vi "Measurement Logic.vi"(8 "error in":errorcluster, 9 "measurement configuration":T2={"TDMS File Path"="", "TDMS Channels"=["", ""], "FGEN Resource Names"=["", ""], "TDMS Groups"=["", ""], "FGEN Waveform Names"=["", ""], "Export Marker0 From File?"=TRUE, "Waveform Sequence"=["", ""], "Loops Sequence"=[]}, 10 "measure call context in":refnum<class "Measure Call Context.lvclass">) -> (0 "error out":errorcluster, 1 "measurement results":T1, 2 "measure call context out":refnum<class "Measure Call Context.lvclass">)   [LabVIEW 2025, in "FGEN Arb Sequence Mode.lvclass"]
doc: "Contains the core logic for executing the measurement."
uses:
  FGEN Arb Sequence Mode.lvclass
  <vilib>/Plug-In SDKs/Measurements/Measure Call Context/Measure Call Context.lvclass
  Measurement Configuration.ctl
  Measurement Results.ctl
  71329b31-811e-493e-9c7a-fa078d8b0f92.vi
  71329b31-811e-493e-9c7a-fa078d8b0f92.vi/9a3a9ab8-4bd1-41e7-91e7-3b9acfe124d7.vi
  <vilib>/Utility/error.llb/Error Cluster From Error Code.vi
  <extravilib>/ChannelInstances/Event Messenger-bool/Instantiate.vi
  FGEN Arb Sequence Mode.lvclass/FGEN Arb Sequence Mode.ctl
  <vilib>/Plug-In SDKs/Clients/Session Management V1/Session Reservation/Session Reservation.lvclass
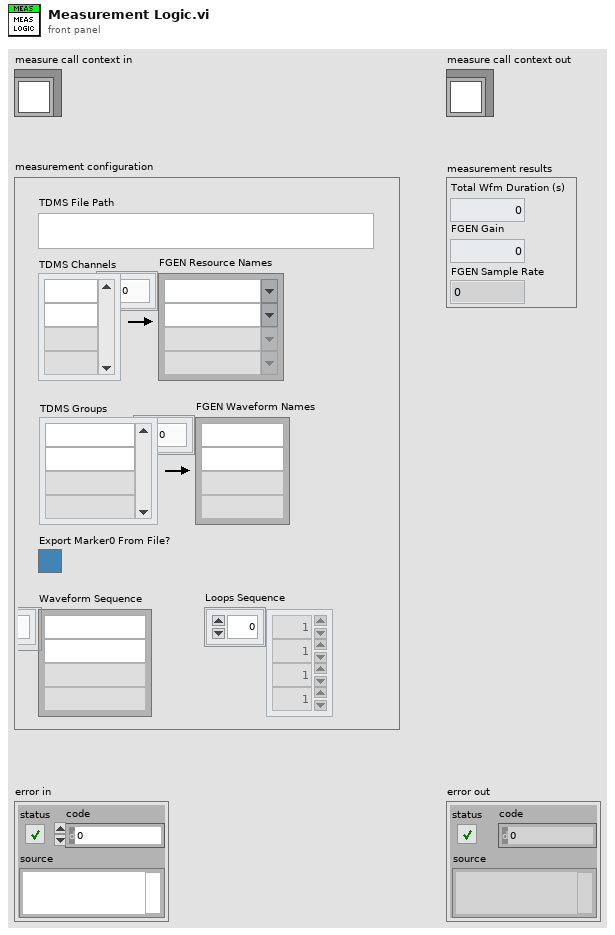
[diagram p1: front panel]
types:
  T1 = typedef "FGEN Arb Sequence Mode.lvclass/Measurement Results.ctl" = cluster{"Total Wfm Duration (s)":dbl, "FGEN Gain":dbl, "FGEN Sample Rate":dbl}
  T2 = typedef "FGEN Arb Sequence Mode.lvclass/Measurement Configuration.ctl" = cluster{"TDMS File Path":string, "TDMS Channels":string[], "FGEN Resource Names":string[], "TDMS Groups":string[], "FGEN Waveform Names":string[], "Export Marker0 From File?":bool, "Waveform Sequence":string[], "Loops Sequence":u32[]}
  T3 = cluster{"FGEN Channels":string[], "FGEN Gain":dbl, "FGEN Wfm Sequence":string[], "FGEN Loops Sequence":u32[], "FGEN Wfm Map":map{string, cluster{"Waveforms":waveform(dbl)[], "Markers":dbl}}, "Sample Rate":dbl}
  T4 = cluster{"FGEN Channel Mapping":string[][], "FGEN Wfm List":string[][]}
  T5 = cluster{"FGEN Channels":string[], "FGEN Gain":dbl, "FGEN Sample Rate":dbl, "FGEN Wfm Map":map{string, cluster{"Waveforms":waveform(dbl)[], "Markers":dbl}}}
  T6 = map{string, cluster{"Waveforms":waveform(dbl)[], "Markers":dbl}}
  T7 = cluster{"session reservation out":refnum<class "Session Reservation.lvclass">, "session":refnum<k15>}
  T8 = typedef "Event Messenger-bool.lvlib/))Channel.ctl" = refnum<queue>
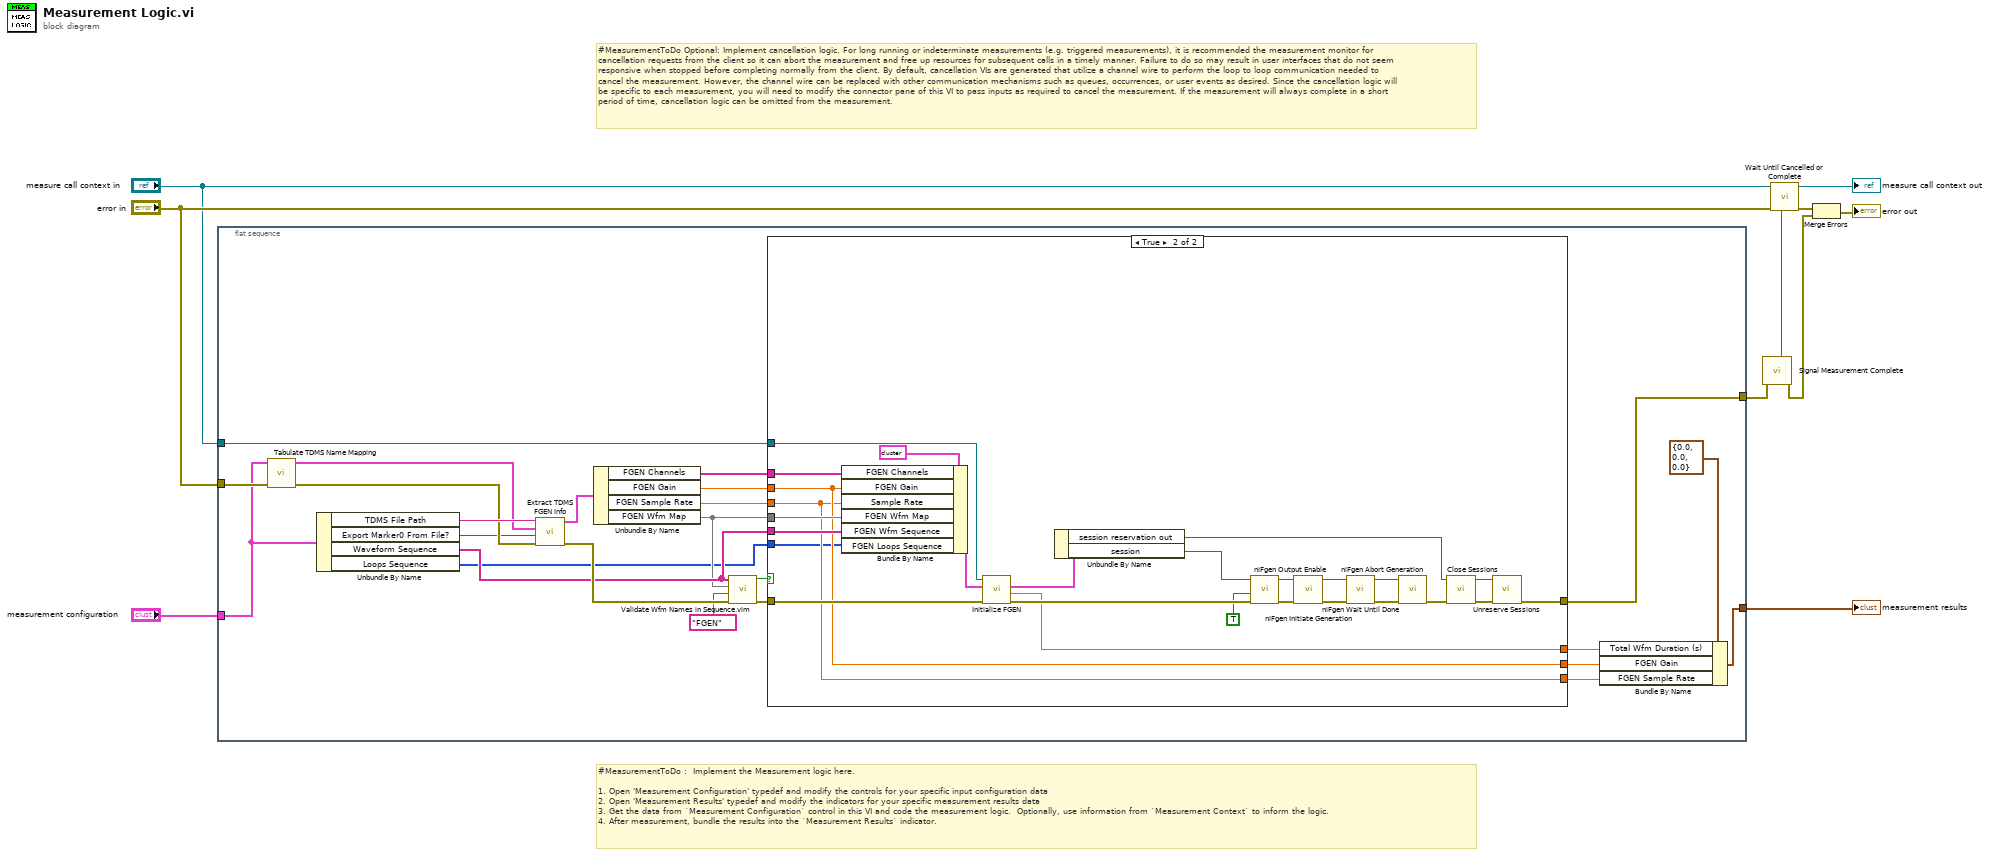
[diagram p0: block diagram]
diagram:
  # "#MeasurementToDo Optional: Implement cancellation logic. For long running or indeterminate measurements (e.g. triggered measurements), it is recommended the measurement monitor for cancellation requests from the client so it can abort the measurement and free up resources for subsequent calls in a timely manner. Failure to do so may result in user interfaces that do not seem responsive when stopped before completing normally from the client. By default, cancellation VIs are generated that utilize a channel wire to perform the loop to loop communication needed to cancel the measurement. However, the channel wire can be replaced with other communication mechanisms such as queues, occurrences, or user events as desired. Since the cancellation logic will be specific to each measurement, you will need to modify the connector pane of this VI to pass inputs as required to cancel the measurement. If the measurement will always complete in a short period of time, cancellation logic can be omitted from the measurement."
  # "#MeasurementToDo :  Implement the Measurement logic here.\n\n1. Open 'Measurement Configuration' typedef and modify the controls for your specific input configuration data\n2. Open 'Measurement Results' typedef and modify the indicators for your specific measurement results data\n3. Get the data from `Measurement Configuration` control in this VI and code the measurement logic.  Optionally, use information from `Measurement Context` to inform the logic.\n4. After measurement, bundle the results into the `Measurement Results` indicator."
  n1 = flat-sequence {
    tunnel: "measurement configuration" -> [w20]
    tunnel: [w33] -> w9
    tunnel: "error in" -> [w28]
    tunnel: [w15] -> w6
    tunnel: "measure call context in" -> [w23]
    frame #0 {
      n2 = call "Tabulate TDMS Name Mapping.vi"("error in"=w28, "measurement configuration"=w20) -> ("error out"=w30:errorcluster, "TDMS Name Mapping"=w31:T4)  [unwired: 8 in]
      n3 = Unbundle By Name(w20) -> ("TDMS File Path"=w32:string, "Export Marker0 From File?"=w27:bool, "Waveform Sequence"=w21:string[], "Loops Sequence"=w11:u32[])
      n4 = call "Extract TDMS FGEN Info.vi"("error in (no error)"=w30, "Export Marker0 From File?"=w27, "TDMS Name Mapping"=w31, "TDMS File Path"=w32) -> ("error out"=w29:errorcluster, "TDMS FGEN Info"=w25:T5)  [unwired: 6 in]
      n5 = Unbundle By Name(w25) -> ("FGEN Channels"=w22:string[], "FGEN Gain"=w17:dbl, "FGEN Sample Rate"=w16:dbl, "FGEN Wfm Map"=w19:T6)
      n6 = call "Validate Wfm Names in Sequence.vim"("error in"=w29, "Wfm Resource Type"="FGEN", "Wfm Map"=w19, "Wfm Sequence"=w21) -> ("error out"=w26:errorcluster, "All Waveform Name Valid?"=w14:bool)  [unwired: 6 in]
      n7 = case shown="True" w14 {
        tunnel: w26 -> [w35 w61]
        tunnel: w23 -> [_ w59]
        tunnel: w22 -> [_ w57]
        tunnel: w21 -> [_ w56]
        tunnel: w19 -> [_ w55]
        tunnel: [_ w53] -> w18
        tunnel: w17 -> [_ w40]
        tunnel: w16 -> [_ w39]
        tunnel: [w35 w46] -> w15
        tunnel: [_ w40] -> w13
        tunnel: [_ w39] -> w12
        tunnel: w11 -> [_ w36]
        frame False {
        }
        frame True {
          n8 = Bundle By Name(cluster=T3 {"FGEN Channels"=[], "FGEN Gain"=0.0, "FGEN Wfm Sequence"=[], "FGEN Loops Sequence"=[], "FGEN Wfm Map"={}, "Sample Rate"=0.0} ("FGEN Settings"), "FGEN Channels"=w57, "FGEN Gain"=w40, "Sample Rate"=w39, "FGEN Wfm Map"=w55, "FGEN Wfm Sequence"=w56, "FGEN Loops Sequence"=w36) -> (w58:T3)
          n9 = call "Initialize FGEN.vi"("error in (no error)"=w61, "FGEN Settings"=w58, "measurement context in"=w59) -> ("error out"=w60:errorcluster, "Total Wfm Duration (s)"=w53:dbl, "FGEN Sessions"=w54:T7)  [unwired: 5 in, 1 out]
          n10 = Unbundle By Name(w54) -> ("session reservation out"=w45:refnum<class "Session Reservation.lvclass">, "session"=w48:refnum<k15>)
          n11 = call <instrlib>:"niFgen Output Enable.vi"("error in (no error)"=w60, "Output Enable (default: True)"=TRUE, "Instrument Handle"=w48) -> ("error out"=w50:errorcluster, "Instrument Handle Out"=w49:refnum<k15>)  [unwired: 7 in]
          n12 = call <instrlib>:"niFgen Initiate Generation.vi"("error in (no error)"=w50, "Instrument Handle"=w49) -> ("error out"=w51:errorcluster, "Instrument Handle Out"=w42:refnum<k15>)  [unwired: 8 in]
          n13 = call <instrlib>:"niFgen Wait Until Done.vi"("error in (no error)"=w51, "Instrument Handle"=w42) -> ("error out"=w43:errorcluster, "Instrument Handle Out"=w41:refnum<k15>)  [unwired: 8 in]
          n14 = call <instrlib>:"niFgen Abort Generation.vi"("error in (no error)"=w43, "Instrument Handle"=w41) -> ("error out"=w52:errorcluster)  [unwired: 8 in, 1 out]
          n15 = call <vilib>:"Close Sessions.vi"("error in"=w52, "session reservation in"=w45) -> ("error out"=w47:errorcluster, "session reservation out"=w44:refnum<class "Session Reservation.lvclass">)  [unwired: 8 in]
          n16 = call <vilib>:"Unreserve Sessions.vi"("error in"=w47, "session reservation in"=w44) -> ("error out"=w46:errorcluster)  [unwired: 9 in]
        }
      }
      n17 = Bundle By Name(cluster=T1 {"Total Wfm Duration (s)"=0.0, "FGEN Gain"=0.0, "FGEN Sample Rate"=0.0} ("Measurement Results"), "Total Wfm Duration (s)"=w18, "FGEN Gain"=w13, "FGEN Sample Rate"=w12) -> (w33:T1)
    }
  }
  n18 = call "Signal Measurement Complete.vi"("error in (no error)"=w6) -> ("error out"=w4:errorcluster, "done channel"=w5:T8)  [unwired: 9 in]
  n19 = call "Wait Until Cancelled or Complete.vi"("done channel"=w5, "error in (no error)"="error in", "measure call context in"="measure call context in") -> ("error out"=w3:errorcluster, "measure call context out"=→"measure call context out":refnum<class "Measure Call Context.lvclass">)  [unwired: 7 in]
  n20 = Merge Errors(w3, w4) -> (→"error out":errorcluster)
  "measurement results" <- w9
